vi "Read Default Value.vi"(8 "error in":errorcluster, 11 "digital channel in":refnum<class "Digital Channel.lvclass">) -> (0 "error out":errorcluster, 2 "default value":bool, 3 "digital channel out":refnum<class "Digital Channel.lvclass">)   [LabVIEW 2020, in "Scan Engine Scripting.lvlib" / "Digital Channel.lvclass"]
uses:
  Digital Channel.lvclass
  Digital Channel.lvclass/Digital Channel.ctl
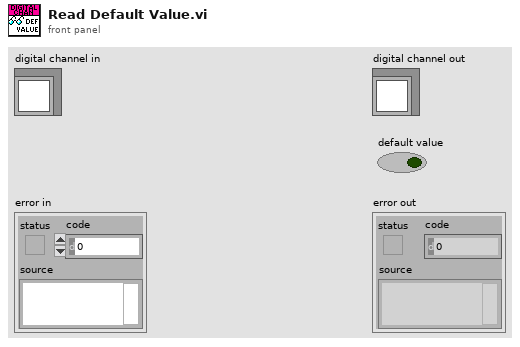
[diagram p1: front panel]
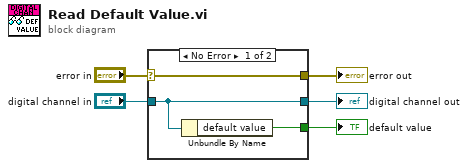
[diagram p0: block diagram]
diagram:
  n1 = case shown="No Error" "error in" {
    selector: "error in" -> [w8 w9]
    tunnel: [w8 w9] -> w4
    tunnel: [w7 w10] -> w2
    tunnel: "digital channel in" -> [w7 w10]
    tunnel: [w6 _] -> w1
    frame No Error {
      n2 = Unbundle By Name(w7) -> ("default value"=w6:bool)
    }
    frame Error {
    }
  }
  "error out" <- w4
  "digital channel out" <- w2
  "default value" <- w1
